vi "En Face Range Selection.vi"(11 "IntensityGraph in":refnum<vi>) -> (2 "Lower En Face":dbl, 3 "Upper En Face":dbl)   [LabVIEW 2014]
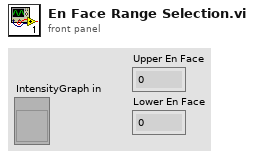
[diagram p1: front panel]
types:
  T1 = typedef "LVCursorListTypeDef.ctl" = cluster{"Name":string, "Color":u32, "Style":u8, "Point Style":u8, "Name Visible":bool, "Allow Drag":bool, "Cursor Mode":u32, "Plot":i32, "Index":i32, "Position":cluster{"X":dbl, "Y":dbl}, "X Scale":u32, "Y Scale":u32, "Watch Plots":i32[], "Watch All Plots":bool, "Plot Area":i32, "Label Offset":cluster{"X":dbl, "Y":dbl}}[]
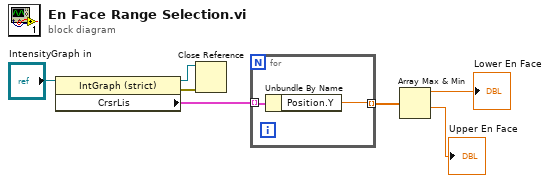
[diagram p0: block diagram]
diagram:
  n1 = property class="IntGraph (strict)"(reference="IntensityGraph in") -> (reference out=w1:refnum<vi>, error out=w2:errorcluster, "CrsrLis"=w6:T1)  [unwired: 1 in]
  n2 = Close Reference(reference=w1, error in (no error)=w2) -> ()  [unwired: 1 out]
  n3 = for {
    tunnel: w6 -> [w9] mode=indexing
    tunnel: [w8] -> w5 mode=indexing
    n4 = Unbundle By Name(w9) -> ("Position.Y"=w8:dbl)
  }
  n5 = Array Max & Min(array=w5) -> (max value=→"Lower En Face":dbl, min value=→"Upper En Face":dbl)  [unwired: 2 out]
